vi "Read Message Stream.vi"(11 "Network Endpoint in":refnum<class "Network Endpoint.lvclass">) -> (2 "Message Stream":refnum<class "Message Stream.lvclass">)   [LabVIEW 2020, in "Network Endpoint.lvlib" / "Network Endpoint.lvclass"]
doc: "Returns the message stream object being used by this endpoint."
uses:
  Network Endpoint.lvclass
  Abstract Classes/Message Stream/Message Stream.lvclass
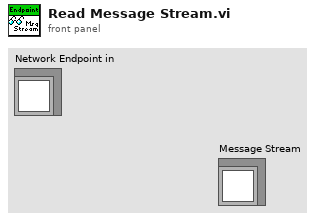
[diagram p1: front panel]
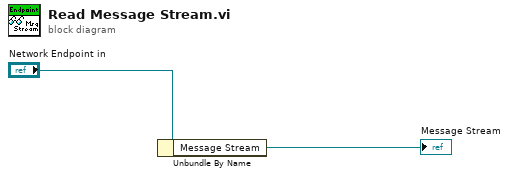
[diagram p0: block diagram]
diagram:
  n1 = Unbundle By Name("Network Endpoint in") -> ("Message Stream"=→"Message Stream":refnum<class "Message Stream.lvclass">)
